vi "Signal Input.vi"(8 "error in (no error)":errorcluster, 9 "Gain":dbl=1.0 format="%_2p", 10 "Signal":dbl format="%_2p") -> (0 "error out":errorcluster)   [LabVIEW 2017, in "Haptic Prog Interface.lvlib"]
doc: "Returns the forces of the haptic pen in N.\n\n<b>Position:</b> Returns a cluster of the x, y, and z forces on the pen (in units of N)."
uses:
  Haptic Prog Interface.lvlib
  Haptic-Programming-Interface/src/x64/Debug/Haptic Programming Interface.dll
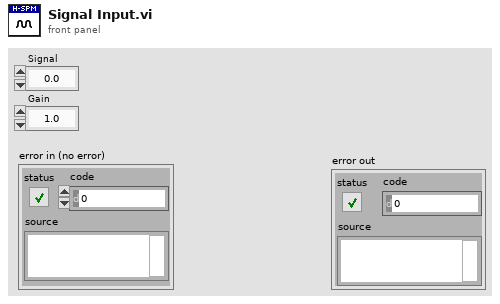
[diagram p1: front panel]
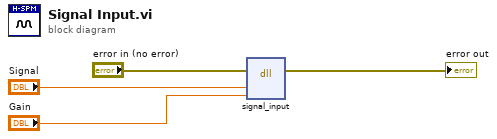
[diagram p0: block diagram]
diagram:
  n1 = dll-call lib="C:/Users/freem/Documents/GitHub/HapticSPM/Haptic-Programming-Interface/src/x64/Debug/Haptic Programming Interface.dll" fn="signal_input"(error in="error in (no error)", "input_signal"="Signal", "input_gain"="Gain") -> (error out=→"error out":errorcluster)  [unwired: 5 in, 1 out]
